vi "Utility MODBUS RTU Send Message.vi"(6 "Command (0)":u8, 7 "Unit Address (1)":u8=1, 8 "error in (no error)":errorcluster, 10 "Message (empty array)":u8[](array[numeric]), 11 "VISA resource name":refnum<visa-resource-name>) -> (0 "error out":errorcluster, 2 "Length Of Sent MSG":u8, 3 "VISA resource name out":refnum<visa-resource-name>)   [LabVIEW 2010]
doc: "This VI sends the MODBUS message."
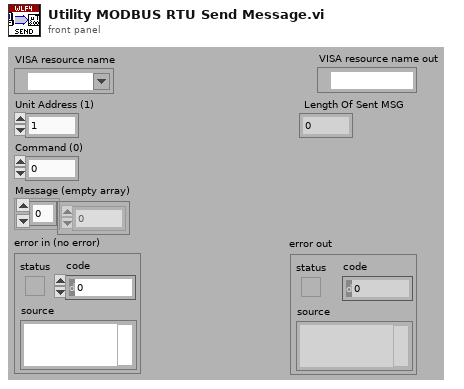
[diagram p1: front panel]
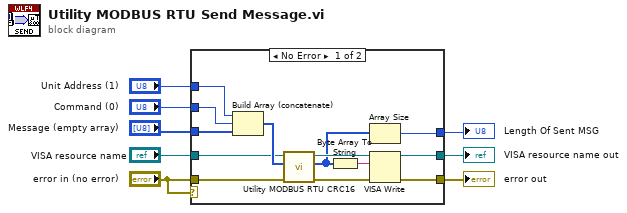
[diagram p0: block diagram]
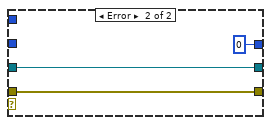
[diagram p2: hidden frame]
diagram:
  n1 = case shown="No Error" "error in (no error)" {
    tunnel: "error in (no error)" -> [w21 w23]
    tunnel: [w19 w23] -> w8
    tunnel: [w18 w24] -> w7
    tunnel: "Command (0)" -> [w17 _]
    tunnel: "Unit Address (1)" -> [w16 _]
    tunnel: "VISA resource name" -> [w13 w24]
    tunnel: [w12 0] -> w3
    tunnel: "Message (empty array)" -> [w10 _]
    frame No Error {
      n2 = Build Array (concatenate)(w16, w17, w10) -> (w14:u8[])
      n3 = call "Utility MODBUS RTU CRC16.vi"("error in (no error)"=w21, "Message (empty array)"=w14, "VISA resource name"=w13) -> ("error out"=w20:errorcluster, "Message with CRC"=w11:u8[], "VISA resource name out"=w15:refnum<visa-resource-name>)  [unwired: 5 in, 1 out]
      n4 = Byte Array To String(unsigned byte array=w11) -> (string=w9:string)
      n5 = Array Size(array=w11) -> (size(s)=w12:i32)
      n6 = VISA Write(VISA resource name=w15, write buffer=w9, error in (no error)=w20) -> (VISA resource name out=w18:refnum<visa-resource-name>, error out=w19:errorcluster)  [unwired: 1 out]
    }
    frame Error {
    }
  }
  "error out" <- w8
  "VISA resource name out" <- w7
  "Length Of Sent MSG" <- w3
